vi "XY Graph 1-Normalize Plot.vi"(8 "error in (no error)":errorcluster, 9 "Replace Plot (T)?":bool=TRUE, 11 "Selected Plot Info":T1={"Multiplot XY Graph"=refnum, "Mouse Coordinates"={"Horizontal"=0, "Vertical"=0}, "Plot Index"=-1}) -> (0 "Error Out":errorcluster, 1 "1-Normalize Plot Message":string, 3 "1-Normalized Plot":cluster{"t Array":dbl[], "IRF Array":dbl[]})   [LabVIEW 2021, in "XY Graph Add-Ons.lvlib"]
uses:
  XY Graph Selected Plot Info.ctl
  XY Graph Refnum.ctl
  <vilib>/Utility/miscctls.llb/LVPoint32TypeDef.ctl
  XY Graph Add-Ons.lvlib
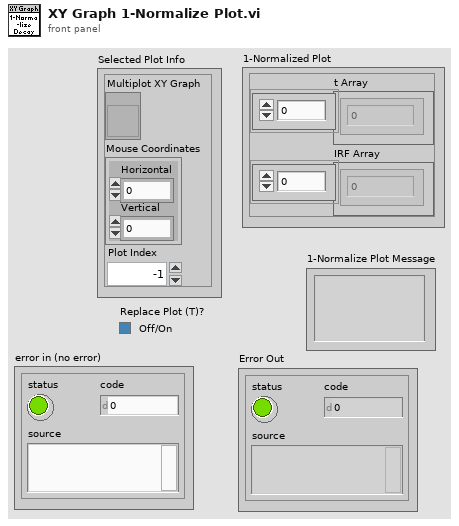
[diagram p1: front panel]
types:
  T1 = typedef "XY Graph Add-Ons.lvlib/XY Graph Selected Plot Info.ctl" = cluster{"Multiplot XY Graph":T2, "Mouse Coordinates":T3, "Plot Index":i32}
  T2 = typedef "XY Graph Add-Ons.lvlib/XY Graph Refnum.ctl" = refnum<vi>
  T3 = typedef "LVPoint32TypeDef.ctl" = cluster{"Horizontal":i32, "Vertical":i32}
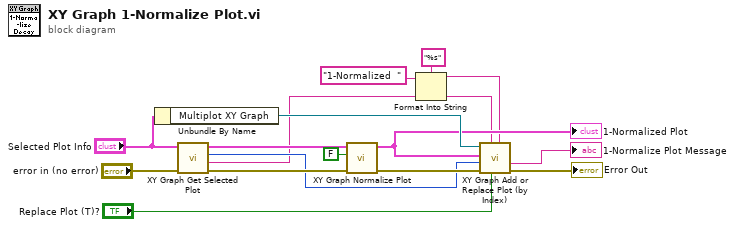
[diagram p0: block diagram]
diagram:
  n1 = Unbundle By Name("Selected Plot Info") -> ("Multiplot XY Graph"=w12:T2)
  n2 = call "XY Graph Get Selected Plot.vi"("error in (no error)"="error in (no error)", "Selected Plot Info"="Selected Plot Info") -> ("error out"=w10:errorcluster, "Plot Name"=w2:string, "Plot Index"=w6:i32, "Plot"=w11:cluster{"X Array":dbl[], "Y Array":dbl[]})  [unwired: 4 in, 2 out]
  n3 = call "XY Graph Normalize Plot.vi"("Error In"=w10, "Subtract Baseline? (No)"=FALSE, "Plot in"=w11) -> ("Error Out"=w9:errorcluster, "Plot out"=w7:cluster{"X Array":dbl[], "Y Array":dbl[]})  [unwired: 7 in]
  "1-Normalized Plot" <- w7
  n4 = Format Into String(format string="%s", initial string="1-Normalized  ", w2) -> (resulting string=w3:string)  [unwired: 1 in, 1 out]
  n5 = call "XY Graph Add or Replace Plot (by Index).vi"("New Plot Name"=w3, "Replace Plot (T)?"="Replace Plot (T)?", "Original Plot Name"=w2, "error in (no error)"=w9, "Plot Index"=w6, "Plot in"=w7, "XYGraph in"=w12) -> ("error out"=→"Error Out":errorcluster, "Message"=→"1-Normalize Plot Message":string)  [unwired: 3 in]
